vi "sub_vi.vi"(1 "B":dbl, 2 "A":dbl) -> (0 "C":dbl)   [LabVIEW 2015]
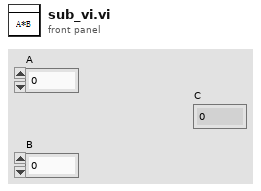
[diagram p1: front panel]
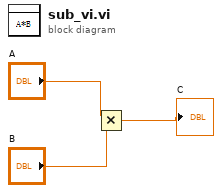
[diagram p0: block diagram]
diagram:
  n1 = Multiply(x="A", y="B") -> (x*y=→"C":dbl)
